vi "Main.vi"() -> ()   [LabVIEW 2019]
uses:
  Support/Gamepad.ctl
  Support/Color.ctl
  Simulation Support/ControlPanel_Picture.ctl
  Simulation Support/Arm_Picture.ctl
  Support/Control Panel Motors.ctl
panel:
  out "ControlPanel Top View":T1
  out "Arm":T2
  out "Arm In":bool
  out "Arm Out":bool
  out "Color":T3
  in  "stop":bool
  in  "Gamepad":T4={"A"=FALSE, "B"=FALSE, "X"=FALSE, "Y"=FALSE, "LB"=FALSE, "RB"=FALSE, "Back"=FALSE, "Next"=FALSE, "Left Stick X"=0.0, "Left Stick Y"=0.0, "Right Stick X"=0.0, "Right Stick Y"=0.0, "LT"=1.0, "RT"=1.0, "D-Pad X"=0, "D-Pad Y"=0} {"Left Stick X" scale=-1.0..1.0; "Left Stick Y" scale=1.0..-1.0; "Right Stick X" scale=-1.0..1.0; "Right Stick Y" scale=1.0..-1.0; "D-Pad Y" step=1 scale=1.0..-1.0; "D-Pad X" step=1 scale=-1.0..1.0; "LT" scale=1.0..-1.0; "RT" scale=1.0..-1.0}
  out "Control Panel Motor":dbl(slide) scale=-1.0..1.0
  out "Arm Motor":dbl(slide) scale=-1.0..1.0
  out "Control Panel Full":dbl
  out "Control Panel":dbl(knob) scale=0.0..1.0
  out "Arm":dbl(knob) scale=0.0..1.0
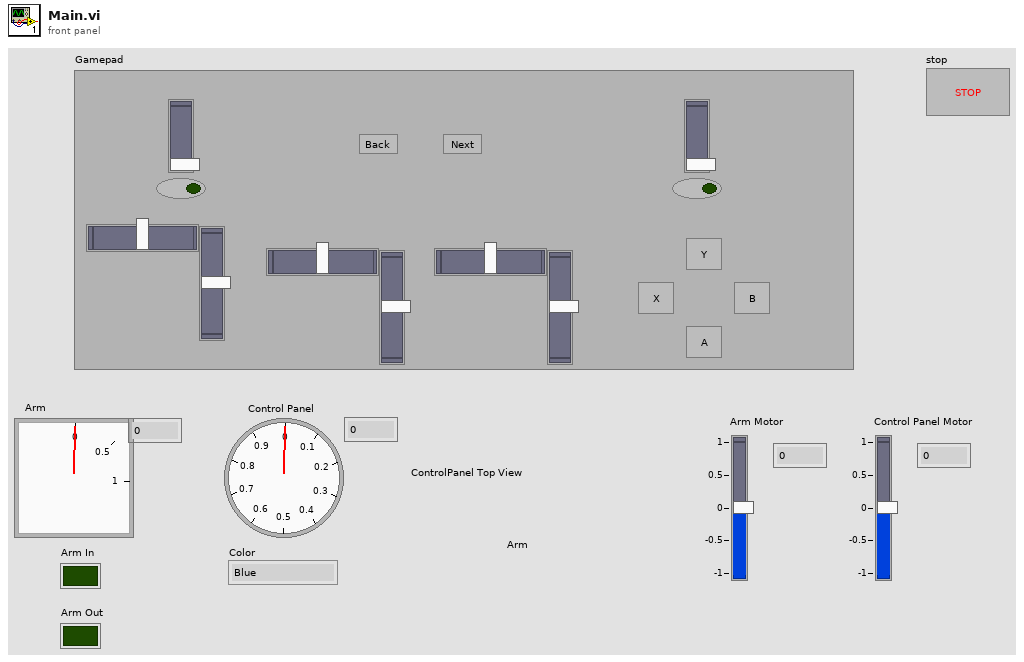
[diagram p1: front panel]
types:
  T1 = typedef "ControlPanel_Picture.ctl" = picture
  T2 = typedef "Arm_Picture.ctl" = picture
  T3 = typedef "Color.ctl" = enum16{"Blue", "Green", "Red", "Yellow"}
  T4 = typedef "Gamepad.ctl" = cluster{"A":bool, "B":bool, "X":bool, "Y":bool, "LB":bool, "RB":bool, "Back":bool, "Next":bool, "Left Stick X":dbl, "Left Stick Y":dbl, "Right Stick X":dbl, "Right Stick Y":dbl, "LT":dbl, "RT":dbl, "D-Pad X":i32, "D-Pad Y":i32}
  T5 = typedef "Control Panel Motors.ctl" = cluster{"Arm":dbl, "Wheel":dbl}
  T6 = typedef "Rotated_Picture_TypeDef.ctl" = cluster{"ONE-8-bit pixmap":u8[][], "Two-Array":cdb[][], "Three-Numeric":i32, "Four-Numeric":i32, "Five-Numeric":cdb, "Six-colors":u32[], "Seven-new element/subarray":u32, "Eight-Cluster":cluster{"[0]":i32, "[1]":i32}}
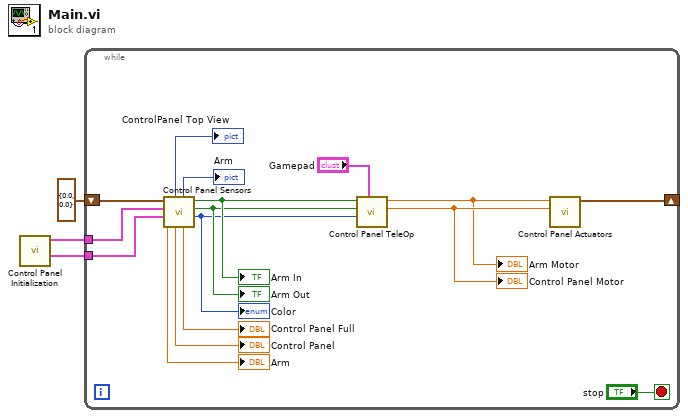
[diagram p0: block diagram]
diagram:
  n1 = call "Control Panel Initialization.vi"() -> ("ArmRotatedPicture"=w1:T6, "ControlPanelRotatedPicture"=w2:T6)  [unwired: 10 in]
  n2 = while {
    shift-right: [w19] -> _
    shift-left: T5 {"Arm"=0.0, "Wheel"=0.0} ("Color Wheel Motors") -> [w18]
    tunnel: w2 -> [w7]
    tunnel: w1 -> [w6]
    stop <- "stop" stop-if-true
    n3 = call "Control Panel Sensors.vi"("ArmRotatedPicture"=w6, "ControlPanelRotatedPicture"=w7, "Control Panel Motors"=w18) -> ("Color"=w15:T3, "Arm Out"=w16:bool, "Arm In"=w17:bool, "Control Panel Full"=→"Control Panel Full":dbl, "ArmPicture"=→"Arm":picture, "Control Panel"=→"Control Panel":dbl, "ControlPanelPicture"=→"ControlPanel Top View":picture, "Arm"=→"Arm":dbl)  [unwired: 1 in]
    "Color" <- w15
    "Arm Out" <- w16
    "Arm In" <- w17
    n4 = call "Control Panel TeleOp.vi"("Gamepad"="Gamepad", "Color"=w15, "Arm Out"=w16, "Arm In"=w17) -> ("Wheel"=w11:dbl, "Arm"=w10:dbl)  [unwired: 6 in]
    "Arm Motor" <- w10
    "Control Panel Motor" <- w11
    n5 = call "Control Panel Actuators.vi"("Wheel"=w11, "Arm"=w10) -> ("Control Panel Motors"=w19:T5)  [unwired: 9 in]
  }
